vi "CV_MOS_Measurement_inclFIT_abhi.vi"() -> ()   [LabVIEW 2010]
uses:
  <vilib>/Utility/file.llb/Write To Spreadsheet File (DBL).vi
  <vilib>/Utility/file.llb/Read From Spreadsheet File (DBL).vi
panel:
  out "error out":errorcluster
  in  "error in":errorcluster
  in  "Instrument Selector":enum16{"HV source", " V source", "Quasi source"}(ring)
  in  "Ramp_rate(0.5 -10V)":dbl(slide)=1.0 min=0.5 max=10.0 step=0.5 scale=0.0..10.0
  out "1/C2":cluster{dbl[], dbl[]}[](graph)
  out "results":string
  out "Oxide Charge Concentration (cm-2)":dbl format="%.2e"
  out "Oxide Thickness (microns)":dbl format="%.2f"
  out "V fb":dbl format="%.2f"
  out "C accumulation":dbl format="%.2p"
  out "C inversion":dbl format="%.2p"
  in  "MIN FIT POINTS (CMS default 5)\nChi²":i32=5
  in  "IGN FIT POINTS (CMS default 5)\nChi²":i32=5
  in  "MINIMUM FIT POINTS (CMS default 10)\nChi²":i32=10
  in  "IGNORE FIT POINTS (CMS default 10)\nChi²":i32=10
  in  "Filename":path
  in  "OBJECT_ID":string="test"
  in  "measurement":string(combo)="CV_MOS"
  in  "Load data from file":bool
  in  "Start voltage":dbl=-10.0
  out "C vs. V":cluster{dbl[], dbl[]}(graph)={[0.0, 5.0, 10.0, 15.0, 20.0, 25.0, 30.0, 35.0, 40.0, 45.0, 50.0, 55.0, 60.0, 65.0, 70.0, 75.0, 80.0, 85.0, 90.0, 95.0, 100.0], [1.8635578976297996e+19, 9.064596143073316e+19, 9.485171736362531e+19, 7.413850691134297e+19, 7.418704610238344e+19, 7.622026879747919e+19, 7.849656372355467e+19, 7.765081845837147e+19, 8.404766788227577e+19, 8.301854428127594e+19, 9.005168717490718e+19, 9.317993657712276e+19, 9.633776152676888e+19, 9.948400550283798e+19, 1.0259628572927422e+20, 1.0638472809757586e+20, 1.1245277238769877e+20, 1.1010496605124031e+20, 1.1656544215003265e+20, 1.1687388308729507e+20, 1.2836032898103964e+20]}
  in  "LCR initialize":T1(tab)
  in  "Voltage Level (V) (5mV)":dbl=0.25 min=0.005 max=20.0 step=0.001 format="%.1p"
  in  "Current Level (A) (100uA)":dbl min=0.0 max=20.0 step=0.01 format="%.4p"
  in  "Frequency Value (Hz) (100KHz)":dbl=100000.0 min=20.0 max=30000000.0 step=1.0 format="%.0p"
  in  "Oscillator Select (T: Voltage)":bool=TRUE
  in  "Auto Level Control (F: Off)":bool=TRUE
  in  "Imp Range (Ohm) (0.0)":dbl min=0.0 max=100000000.0 step=1.0 format="%.4f"
  in  "Auto Range (F: Off)":bool=TRUE
  in  "Imp Type (0: CPD)":u32(ring)=3 items=["CPD", "CPQ", "CPG", "CPRP", "CSD", "CSQ", "CSRS", "LPQ", "LPD", "LPG", "LPRP", "LSD", "LSQ", "LSRS", "RX", "ZTD", "ZTR", "GB", "YTD", "YTR"]
  in  "Display Page (0: Measurement)":u32(ring) items=["Measurement", "Bin Number", "Bin Count", "List", "Measurement Setup", "Correction Setup", "Limit Table", "List Setup", "System", "Catalog", "SelfTest", "Line String"]
  in  "Cont (F: Off)":bool
  in  "Trigger Source (0: Internal)":u32(slide)=2 max=3 step=1
  in  "Delay Value (s) (0.0)":dbl min=0.0 max=6.0 step=0.1 format="%.4f"
  in  "Averaging Rate (1)":i16(slide)=1 min=1 max=16 scale=1.0..16.0
  in  "Integ Time (0: Short)":u32(slide)=2 max=2 step=1
  out "Secondary Value":dbl=41910.9 format="%.4p"
  out "Capacitance Cp[F]":dbl=8.82642e-11 format="%.4p"
  out "Data Status":bool=TRUE
  in  "Instrument Selector LCR":T2(ring)
  out "Voltage [V]":dbl=100.0 format="%#_3p"
  in  "abort measurement":bool
  in  "Save in File":bool=TRUE
  in  "Wait [ms]":dbl=500.0
  in  "Compliance [uA]":dbl=10.0 format="%.0p"
  in  "Stepsize [V]":dbl=1.0 format="%.1f"
  in  "Voltage Max [V]":dbl=15.0
  # "Einstellungen\nFreq.:75k\nSignal.:100mV\nCPRP\nTRIGGER:BUS\nIntegTime:LONG"
  # "On\nOff"
  # "Internal\nExternal\nBus\nHold"
  # "On\nOff"
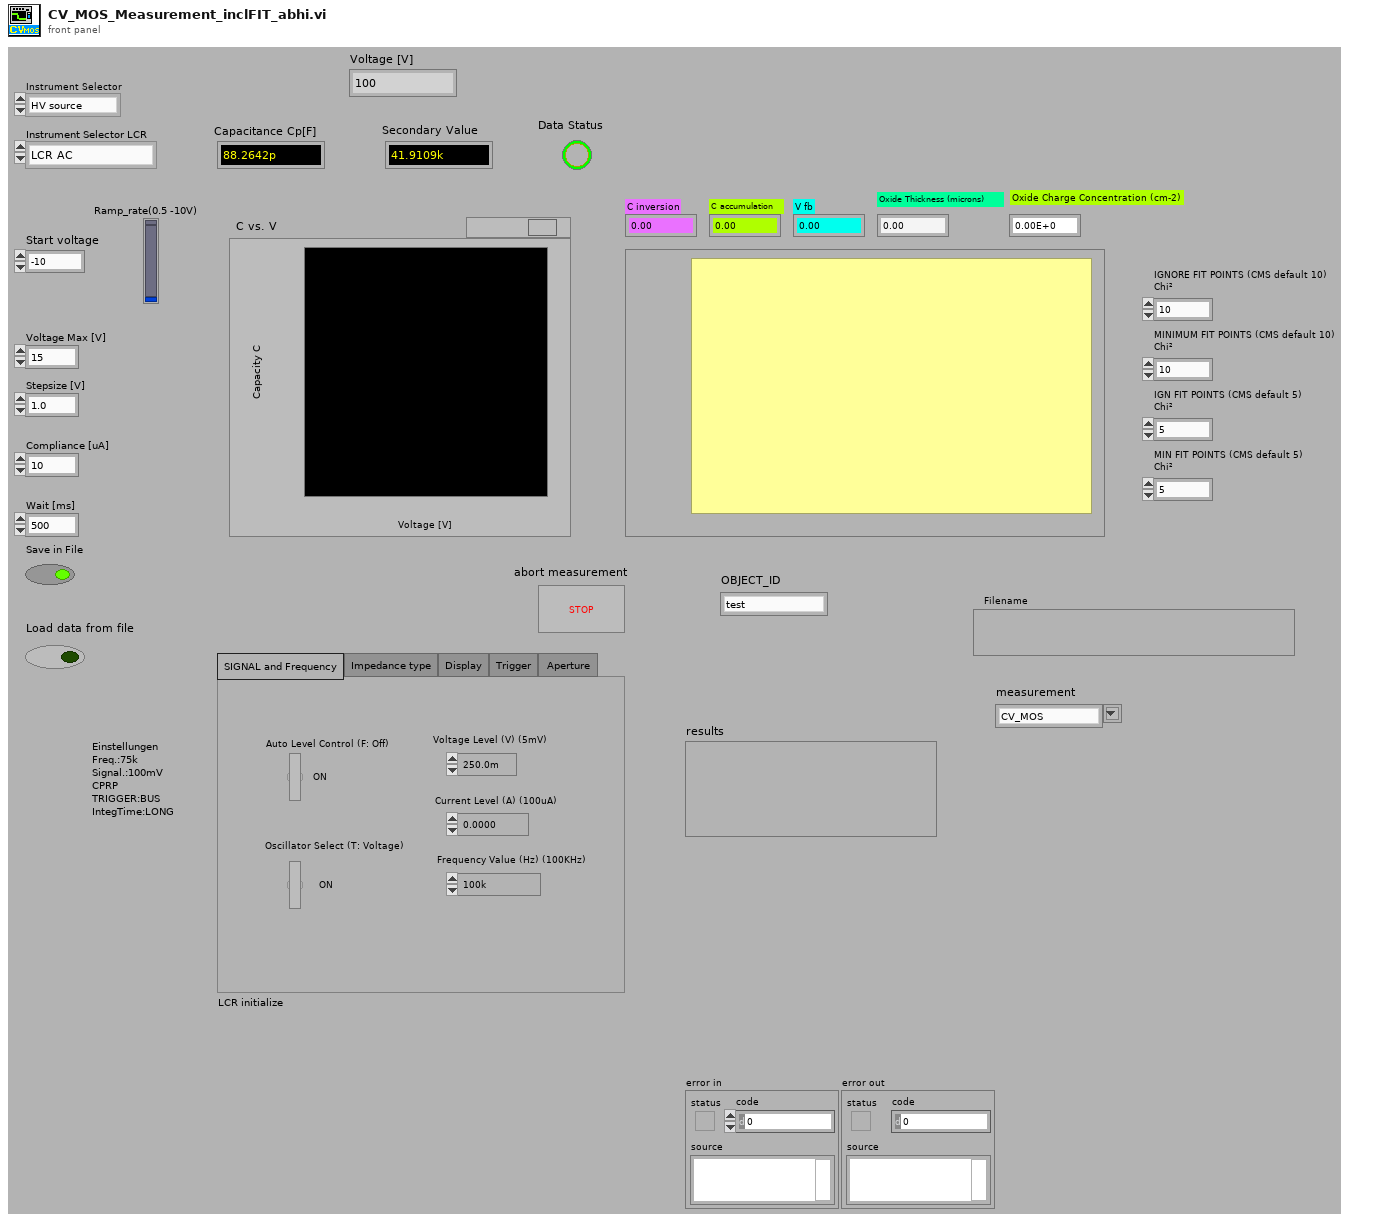
[diagram p1: front panel]
types:
  T1 = enum32{"SIGNAL and Frequency", "Impedance type", "Display", "Trigger", "Aperture "}
  T2 = enum16{"LCR AC", "LCR quasistatic", "old LCR (Karlsruhe)"}
  T3 = cluster{"IGNORE FIT POINTS (CMS default 10)\nChi²":i32, "MINIMUM FIT POINTS (CMS default 10)\nChi²":i32, "IGN FIT POINTS (CMS default 5)\nChi²":i32, "MIN FIT POINTS (CMS default 5)\nChi²":i32}
  T4 = cluster{"Frequency Value (Hz) (100KHz)":dbl, "Current Level (A) (100uA)":dbl, "Auto Level Control (F: Off)":bool, "Voltage Level (V) (5mV)":dbl, "Oscillator Select (T: Voltage)":bool, "Auto Range (F: Off)":bool, "Imp Range (Ohm) (0.0)":dbl, "Imp Type (0: CPD)":u32, "Delay Value (s) (0.0)":dbl, "Display Page (0: Measurement)":u32, "Trigger Source (0: Internal)":u32, "Integ Time (0: Short)":u32, "Cont (F: Off)":bool, "Averaging Rate (1)":i16}
  T5 = cluster{"current [A]":dbl, "voltage [V]":dbl, "compliance reached?":bool, "Primary Value":dbl, "Secondary Value":dbl}
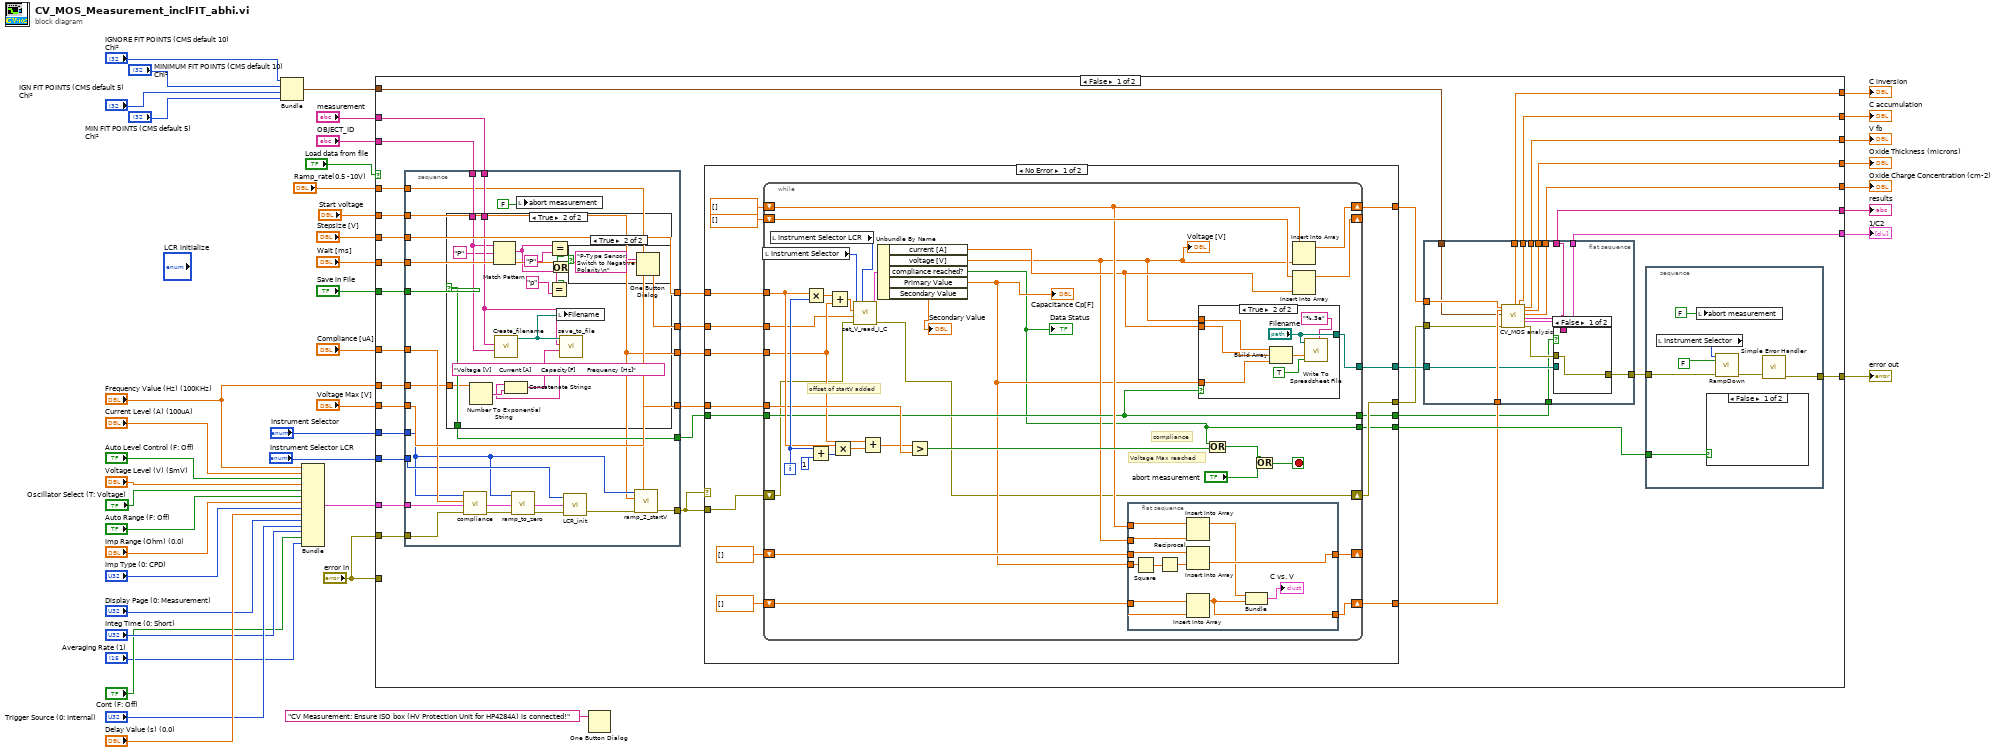
[diagram p0: block diagram]
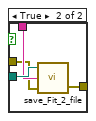
[diagram p2: hidden frame]
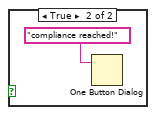
[diagram p3: hidden frame]
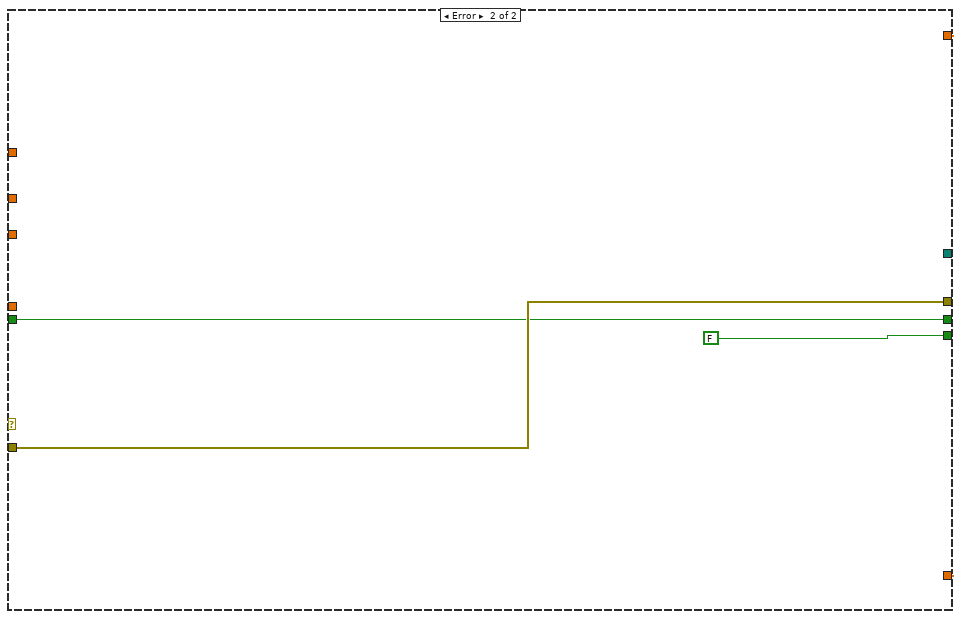
[diagram p5: hidden frame]
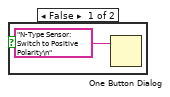
[diagram p7: hidden frame]
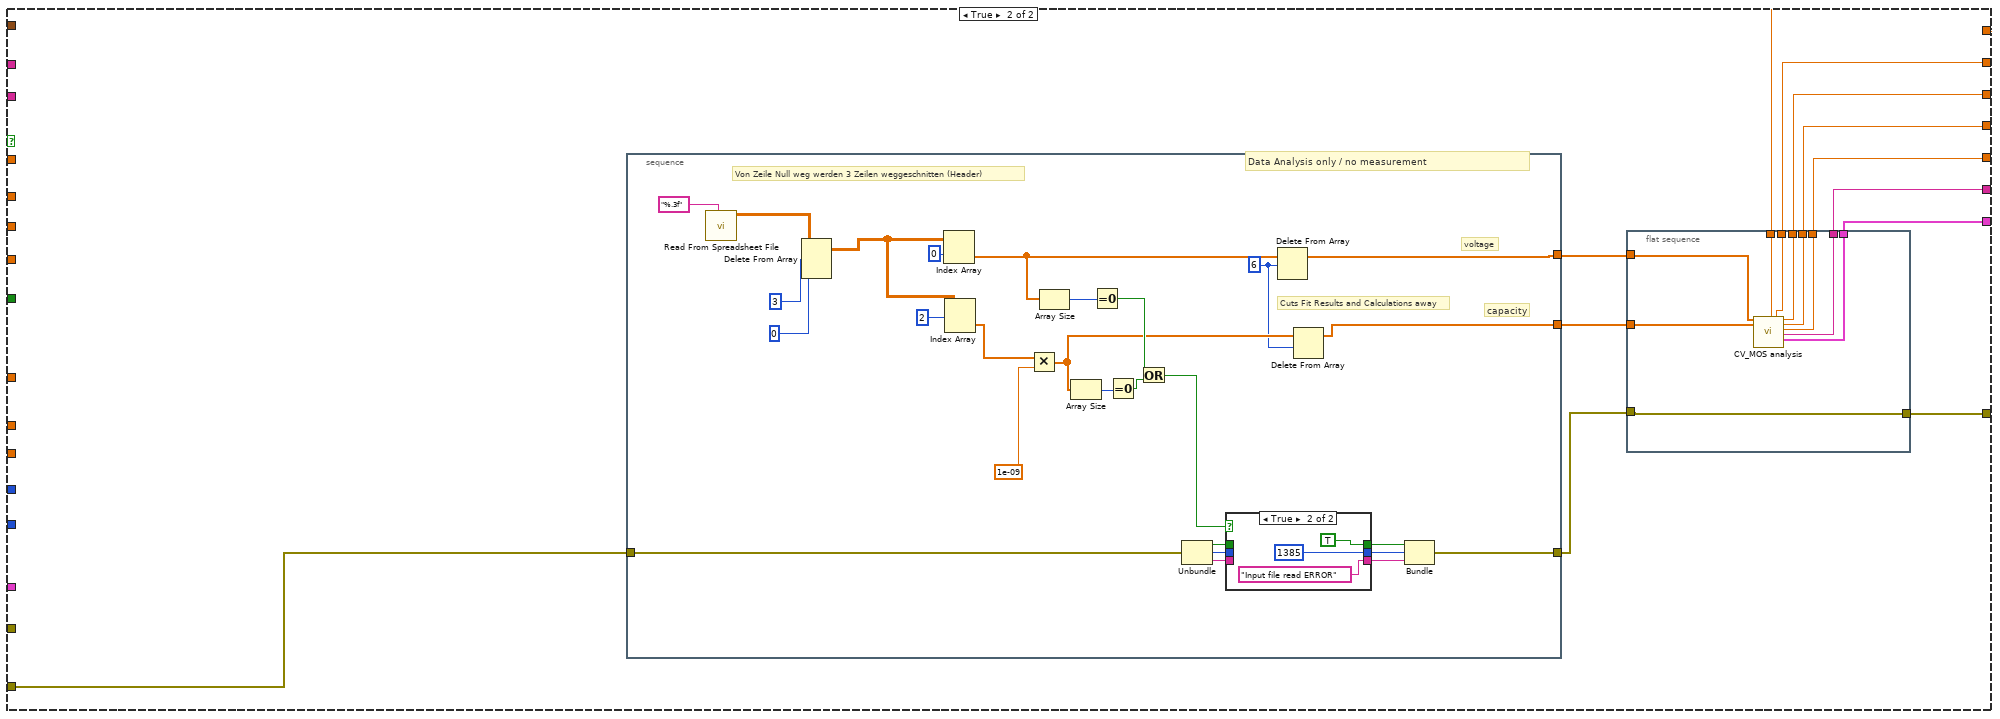
[diagram p8: hidden frame]
diagram:
  n1 = Bundle("IGNORE FIT POINTS (CMS default 10)\nChi²"="IGNORE FIT POINTS (CMS default 10)\nChi²", "MINIMUM FIT POINTS (CMS default 10)\nChi²"="MINIMUM FIT POINTS (CMS default 10)\nChi²", "IGN FIT POINTS (CMS default 5)\nChi²"="IGN FIT POINTS (CMS default 5)\nChi²", "MIN FIT POINTS (CMS default 5)\nChi²"="MIN FIT POINTS (CMS default 5)\nChi²") -> (w5:T3)  [unwired: 1 in]
  n2 = Bundle("Frequency Value (Hz) (100KHz)"="Frequency Value (Hz) (100KHz)", "Current Level (A) (100uA)"="Current Level (A) (100uA)", "Auto Level Control (F: Off)"="Auto Level Control (F: Off)", "Voltage Level (V) (5mV)"="Voltage Level (V) (5mV)", "Oscillator Select (T: Voltage)"="Oscillator Select (T: Voltage)", "Auto Range (F: Off)"="Auto Range (F: Off)", "Imp Range (Ohm) (0.0)"="Imp Range (Ohm) (0.0)", "Imp Type (0: CPD)"="Imp Type (0: CPD)", "Delay Value (s) (0.0)"="Delay Value (s) (0.0)", "Display Page (0: Measurement)"="Display Page (0: Measurement)", "Trigger Source (0: Internal)"="Trigger Source (0: Internal)", "Integ Time (0: Short)"="Integ Time (0: Short)", "Cont (F: Off)"="Cont (F: Off)", "Averaging Rate (1)"="Averaging Rate (1)") -> (w17:T4)  [unwired: 1 in]
  n3 = case shown="False" "Load data from file" {
    tunnel: "Stepsize [V]" -> [w78 _]
    tunnel: "Compliance [uA]" -> [w77 _]
    tunnel: "Wait [ms]" -> [w75 _]
    tunnel: "Save in File" -> [w73 _]
    tunnel: "Voltage Max [V]" -> [w72 _]
    tunnel: "Instrument Selector LCR" -> [w67 _]
    tunnel: "Start voltage" -> [w66 _]
    tunnel: "measurement" -> [w64 _]
    tunnel: "OBJECT_ID" -> [w62 _]
    tunnel: [w61 w230] -> w32
    tunnel: [w60 w229] -> w31
    tunnel: [w59 w228] -> w30
    tunnel: [w58 w227] -> w29
    tunnel: [w57 w226] -> w28
    tunnel: [w52 w225] -> w25
    tunnel: [w56 w224] -> w27
    tunnel: "Ramp_rate(0.5 -10V)" -> [w55 _]
    tunnel: "Instrument Selector" -> [w49 _]
    tunnel: w17 -> [w47 _]
    tunnel: w5 -> [w46 _]
    tunnel: "error in" -> [w45 _]
    tunnel: "error in" -> [_ w221]
    tunnel: [w44 w220] -> w3
    tunnel: "Frequency Value (Hz) (100KHz)" -> [w43 _]
    frame False {
      n4 = stacked-sequence {
        tunnel: [w200] -> w76
        tunnel: w78 -> [w200]
        tunnel: w77 -> [w193]
        tunnel: w75 -> [w199]
        tunnel: [w199] -> w74
        tunnel: w73 -> [w198]
        tunnel: w72 -> [w197]
        tunnel: [w197] -> w71
        tunnel: [w196] -> w70
        tunnel: [w192] -> w69
        tunnel: w67 -> [w189]
        tunnel: w66 -> [w183]
        tunnel: [w183] -> w65
        tunnel: w64 -> [w191]
        tunnel: w62 -> [w190]
        tunnel: w55 -> [w184]
        tunnel: w49 -> [w185]
        tunnel: w47 -> [w186]
        tunnel: w45 -> [w182]
        tunnel: w43 -> [w181]
        frame #0 {
          n5 = case shown="True" w198 {
            selector: w198 -> [w201 w216]
            tunnel: [w201 w216] -> w196
            tunnel: w191 -> [_ w214]
            tunnel: w190 -> [_ w209]
            tunnel: w181 -> [_ w213]
            frame False {
            }
            frame True {
              n6 = Number To Exponential String(number=w213) -> (E-format string=w212:string)  [unwired: 3 in]
              n7 = Match Pattern(string=w209, regular expression="P") -> (match substring=w206:string)  [unwired: 1 in, 3 out]
              n8 = call "Create_filename.vi"("OBJECT_ID"=w209, "measurement"=w214) -> ("filename"=w215:path)  [unwired: 8 in, 1 out]
              n9 = Concatenate Strings("Voltage [V]    Current [A]     Capacity[F]      Frequency [Hz]", w212) -> (w210:string)
              n10 = Equal?(x=w206, y="p") -> (x = y?=w204:bool)
              n11 = Equal?(x=w206, y="P") -> (x = y?=w205:bool)
              n12 = Or(x=w205, y=w204) -> (x .or. y?=w203:bool)
              n13 = local write "Filename"(w215) -> ()
              n14 = call "save_to_file.vi"("Header1"=w210, "HEADER"=w214, "Filename"=w215) -> ()  [unwired: 9 in]
              n15 = case shown="True" w203 {
                frame False {
                  n16 = One Button Dialog(message="N-Type Sensor: Switch to Positive Polarity\n") -> ()  [unwired: 1 in, 1 out]
                }
                frame True {
                  n17 = One Button Dialog(message="P-Type Sensor: Switch to Negative Polarity\n") -> ()  [unwired: 1 in, 1 out]
                }
              }
            }
          }
          n18 = call "compliance.vi"("error in"=w182, "Compliance [A]"=w193, "Instrument Selector"=w185) -> ("error out"=w194:errorcluster)  [unwired: 8 in]
          n19 = call "ramp_to_zero.vi"("error in"=w194, "Instrument Selector"=w185) -> ("error out"=w188:errorcluster)  [unwired: 9 in]
          n20 = local write "abort measurement"(FALSE ("abort measurement")) -> ()
          n21 = call "LCR_init.vi"("error in"=w188, "Cluster"=w186, "Instrument Selector LCR"=w189) -> ("error out"=w187:errorcluster)  [unwired: 1 in]
          n22 = call "ramp_2_startV.vi"("Ramp_rate(0.5 -10V)"=w184, "error in"=w187, "Start voltage"=w183, "Instrument Selector"=w185) -> ("error out"=w192:errorcluster)  [unwired: 7 in]
        }
      }
      n23 = case shown="No Error" w69 {
        tunnel: w76 -> [w122 _]
        tunnel: w74 -> [w121 _]
        tunnel: [w118 w180] -> w51
        tunnel: w71 -> [w117 _]
        tunnel: w70 -> [w116 w176]
        tunnel: w69 -> [w115 w180]
        tunnel: [w114 FALSE ("compliance")] -> w68
        tunnel: w65 -> [w111 _]
        tunnel: [w110 dbl[] []] -> w63
        tunnel: [w109 dbl[] []] -> w54
        tunnel: [w108 _] -> w53
        tunnel: [w107 w176] -> w48
        frame No Error {
          n24 = while {
            tunnel: w116 -> [w135]
            tunnel: w117 -> [w151]
            shift-left: dbl[] [] -> [w145]
            shift-right: [w156] -> w109
            shift-left: dbl[] [] -> [w146]
            shift-right: [w157] -> _
            tunnel: w121 -> [w129]
            tunnel: w122 -> [w153]
            tunnel: [w123] -> w114
            shift-right: [w143] -> _
            shift-left: dbl[] [] ("Capacity") -> [w144]
            shift-right: [w142] -> w110
            shift-left: dbl[] [] -> [w141]
            tunnel: w111 -> [w137]
            tunnel: [w136] -> w108
            tunnel: [w135] -> w107
            shift-right: [w124] -> w118
            shift-left: w115 -> [w125]
            i -> [w155]
            stop <- w148 stop-if-true
            # "offset of startV added"
            # "compliance"
            # "Voltage Max reached"
            n25 = local read "Instrument Selector"() -> (w127:enum16{"HV source", " V source", "Quasi source"})
            n26 = local read "Instrument Selector LCR"() -> (w126:T2)
            n27 = Multiply(x=w153, y=w155) -> (x*y=w140:dbl)
            n28 = Add(x=w155, y=1) -> (x+y=w152:i32)
            n29 = Add(x=w140, y=w137) -> (x+y=w128:dbl)
            n30 = Multiply(x=w153, y=w152) -> (x*y=w138:dbl)
            n31 = call "set_V_read_I_C.vi"("Instrument Selector LCR"=w126, "error in"=w125, "Wait [ms]"=w129, "VoltageLevel"=w128, "Instrument Selector"=w127) -> ("error out"=w124:errorcluster, "output cluster"=w134:T5)  [unwired: 5 in]
            n32 = Add(x=w137, y=w138) -> (x+y=w139:dbl)
            n33 = Unbundle By Name(w134) -> ("current [A]"=w133:dbl, "voltage [V]"=w132:dbl, "compliance reached?"=w123:bool, "Primary Value"=w131:dbl, "Secondary Value"=→"Secondary Value":dbl)
            "Voltage [V]" <- w132
            "Data Status" <- w123
            "Capacitance Cp[F]" <- w131
            n34 = Greater?(x=w139, y=w151) -> (0:w149:bool)
            n35 = flat-sequence {
              tunnel: w145 -> [w167]
              tunnel: w144 -> [w166]
              tunnel: [w165] -> w143
              tunnel: [w162] -> w142
              tunnel: w141 -> [w161]
              tunnel: w132 -> [w159]
              tunnel: w131 -> [w158]
              frame #0 {
                n36 = Square(x=w158) -> (x^2=w164:dbl)
                n37 = Reciprocal(x=w164) -> (1/x=w168:dbl)
                n38 = Insert Into Array(array=w167, new element=w159) -> (w163:dbl[])  [unwired: 1 in]
                n39 = Insert Into Array(array=w166, new element=w168) -> (w165:dbl[])  [unwired: 1 in]
                n40 = Insert Into Array(array=w161, new element=w158) -> (w162:dbl[])  [unwired: 1 in]
                n41 = Bundle(w163, w162) -> (→"C vs. V":cluster{dbl[], dbl[]})  [unwired: 1 in]
              }
            }
            n42 = case shown="True" w135 {
              tunnel: w133 -> [_ w170]
              tunnel: w132 -> [_ w173]
              tunnel: w131 -> [_ w169]
              tunnel: [_ "Filename"] -> w136
              frame False {
              }
              frame True {
                n43 = Build Array(w173, w170, w169) -> (w174:dbl[])
                n44 = call-poly <vilib>:"Write To Spreadsheet File.vi"("format (%.3f)"="%.3e", "append to file? (new file:F)"=TRUE, "1D data"=w174, "file path (dialog if empty)"="Filename") -> ()  [unwired: 4 in, 1 out]
              }
            }
            n45 = Or(x=w123, y=w149) -> (x .or. y?=w150:bool)
            n46 = Or(x=w150, y="abort measurement") -> (x .or. y?=w148:bool)
            n47 = Insert Into Array(array=w145, new element=w132) -> (w156:dbl[])  [unwired: 1 in]
            n48 = Insert Into Array(array=w146, new element=w133) -> (w157:dbl[])  [unwired: 1 in]
          }
        }
        frame Error {
        }
      }
      n49 = flat-sequence {
        tunnel: w51 -> [w91]
        tunnel: w54 -> [w93]
        tunnel: w63 -> [w92]
        tunnel: [w90] -> w61
        tunnel: [w89] -> w60
        tunnel: [w88] -> w59
        tunnel: [w87] -> w58
        tunnel: [w86] -> w57
        tunnel: [w85] -> w56
        tunnel: w53 -> [w84]
        tunnel: [w83] -> w52
        tunnel: [w81] -> w50
        tunnel: w48 -> [w80]
        tunnel: w46 -> [w79]
        frame #0 {
          n50 = call "CV_MOS analysis.vi"("Voltage"=w93, "Capacity"=w92, "Fitparameter_Cluster"=w79, "error in"=w91) -> ("C inversion"=w90:dbl, "C accumulation"=w89:dbl, "V fb"=w88:dbl, "Oxide Thickness (microns)"=w87:dbl, "Oxide Charge Concentration (cm-2)"=w86:dbl, "results"=w83:string, "1/C2"=w85:cluster{dbl[], dbl[]}[], "error out"=w82:errorcluster)  [unwired: 8 in]
          n51 = case shown="False" w80 {
            tunnel: w84 -> [_ w98]
            tunnel: w83 -> [_ w97]
            tunnel: w82 -> [w94 w96]
            tunnel: [w94 w95] -> w81
            frame False {
            }
            frame True {
              n52 = call "save_Fit_2_file.vi"("error in"=w96, "results"=w97, "Filename"=w98) -> ("error out"=w95:errorcluster)  [unwired: 1 in]
            }
          }
        }
      }
      n53 = stacked-sequence {
        tunnel: w68 -> [w103]
        tunnel: w50 -> [w102]
        tunnel: [w99] -> w44
        frame #0 {
          n54 = local read "Instrument Selector"() -> (w101:enum16{"HV source", " V source", "Quasi source"})
          n55 = local write "abort measurement"(FALSE ("abort measurement")) -> ()
          n56 = case shown="False" w103 {
            frame False {
            }
            frame True {
              n57 = One Button Dialog(message="compliance reached!") -> ()  [unwired: 1 in, 1 out]
            }
          }
          n58 = call "RampDown.vi"("error in"=w102, "On/Off"=FALSE, "Instrument Selector"=w101) -> ("error out"=w100:errorcluster)  [unwired: 6 in]
          n59 = call <vilib>:"Simple Error Handler.vi"("error in (no error)"=w100) -> ("error out"=w99:errorcluster)  [unwired: 4 in, 4 out]
        }
      }
    }
    frame True {
      # "Data Analysis only / no measurement"
      n60 = stacked-sequence {
        tunnel: [w234] -> w222
        tunnel: [w233] -> w223
        tunnel: w221 -> [w232]
        tunnel: [w231] -> w219
        frame #0 {
          w237 = 6 ("length")
          # "Cuts Fit Results and Calculations away"
          # "capacity"
          # "voltage"
          # "Von Zeile Null weg werden 3 Zeilen weggeschnitten (Header)"
          n61 = call-poly <vilib>:"Read From Spreadsheet File.vi"("format (%.3f)"="%.3f") -> ("all rows"=w256:dbl[][])  [unwired: 6 in, 4 out]
          n62 = Delete From Array(array=w256, length=3, index (row)=0 ("Disabled Index (col)")) -> (array with subset deleted=w251:dbl[][])  [unwired: 1 in, 1 out]
          n63 = Index Array(array=w251, index (col)=0 ("disabled index (col)")) -> (element=w235:dbl[])  [unwired: 1 in]
          n64 = Index Array(array=w251, index (col)=2 ("disabled index (col)")) -> (element=w236:dbl[])  [unwired: 1 in]
          n65 = Multiply(x=w236, y=1e-09) -> (x*y=w238:dbl[])
          n66 = Array Size(array=w235) -> (size(s)=w248:i32)
          n67 = Array Size(array=w238) -> (size(s)=w249:i32)
          n68 = Equal To 0?(x=w248) -> (x = 0?=w246:bool)
          n69 = Equal To 0?(x=w249) -> (x = 0?=w247:bool)
          n70 = Or(x=w246, y=w247) -> (x .or. y?=w239:bool)
          n71 = Unbundle(w232) -> ("status"=w245:bool, "code"=w243:i32, "source"=w241:string)
          n72 = case shown="True" w239 {
            tunnel: w245 -> [w260 _]
            tunnel: [w260 TRUE ("status")] -> w244
            tunnel: w243 -> [w259 _]
            tunnel: [w259 1385 ("code")] -> w242
            tunnel: w241 -> [w258 _]
            tunnel: [w258 "Input file read ERROR" ("source")] -> w240
            frame False {
            }
            frame True {
            }
          }
          n73 = Delete From Array(array=w235, length=w237) -> (array with subset deleted=w234:dbl[])  [unwired: 1 in, 1 out]
          n74 = Delete From Array(array=w238, length=w237) -> (array with subset deleted=w233:dbl[])  [unwired: 1 in, 1 out]
          n75 = Bundle("status"=w244, "code"=w242, "source"=w240) -> (w231:errorcluster)  [unwired: 1 in]
        }
      }
      n76 = flat-sequence {
        tunnel: [w273] -> w230
        tunnel: [w272] -> w229
        tunnel: [w271] -> w228
        tunnel: [w270] -> w227
        tunnel: [w269] -> w226
        tunnel: [w268] -> w225
        tunnel: [w267] -> w224
        tunnel: w223 -> [w266]
        tunnel: w222 -> [w265]
        tunnel: w219 -> [w264]
        tunnel: [w264] -> w220
        frame #0 {
          n77 = call "CV_MOS analysis.vi"("Voltage"=w265, "Capacity"=w266) -> ("C inversion"=w273:dbl, "C accumulation"=w272:dbl, "V fb"=w271:dbl, "Oxide Thickness (microns)"=w270:dbl, "Oxide Charge Concentration (cm-2)"=w269:dbl, "results"=w268:string, "1/C2"=w267:cluster{dbl[], dbl[]}[])  [unwired: 10 in, 1 out]
        }
      }
    }
  }
  "C inversion" <- w32
  "C accumulation" <- w31
  "V fb" <- w30
  "results" <- w25
  "Oxide Charge Concentration (cm-2)" <- w28
  "Oxide Thickness (microns)" <- w29
  "1/C2" <- w27
  "error out" <- w3
  n78 = One Button Dialog(message="CV Measurement: Ensure ISO box (HV Protection Unit for HP4284A) is connected!") -> ()  [unwired: 1 in, 1 out]
